vi "Shift GPS Output.vi"(1 "GPS Input":cluster{"X pos":i32, "Y pos":i32, "Heading":dbl}) -> (0 "GPS Output":cluster{"X pos":i32, "Y pos":i32, "Heading":dbl})   [LabVIEW 2014]
panel:
  out "Abs Angle":dbl
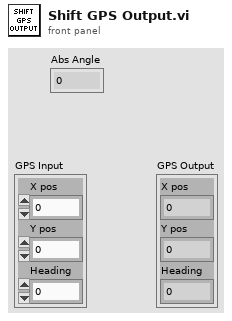
[diagram p1: front panel]
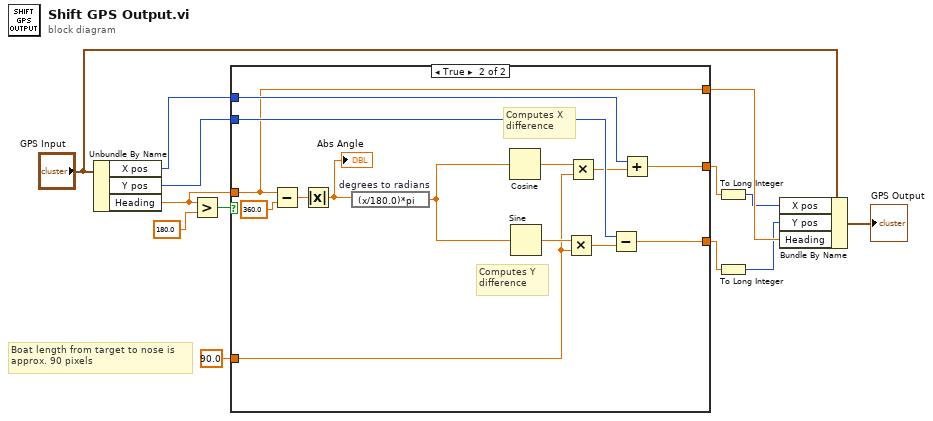
[diagram p0: block diagram]
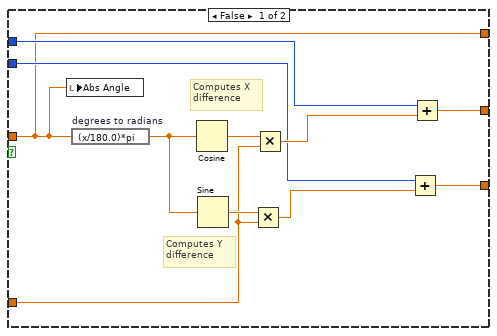
[diagram p2: hidden frame]
diagram:
  # "Boat length from target to nose is \napprox. 90 pixels"
  n1 = Unbundle By Name("GPS Input") -> ("X pos"=w11:i32, "Y pos"=w10:i32, "Heading"=w8:dbl)
  n2 = Greater?(x=w8, y=180.0) -> (0:w12:bool)
  n3 = case shown="True" w12 {
    tunnel: w11 -> [w20 w33]
    tunnel: w10 -> [w18 w32]
    tunnel: 90.0 -> [w22 w34]
    tunnel: w8 -> [w15 w29]
    tunnel: [w17 w31] -> w7
    tunnel: [w16 w30] -> w6
    tunnel: [w15 w29] -> w4
    frame False {
      # "Computes Y \ndifference"
      # "Computes X \ndifference"
      n4 = local write "Abs Angle"(w15) -> ()
      n5 = expression code="(x/180.0)*pi" "degrees to radians"(w15) -> (w14:dbl)
      n6 = Cosine(x=w14) -> (cos(x)=w24:dbl)
      n7 = Sine(x=w14) -> (sin(x)=w23:dbl)
      n8 = Multiply(x=w23, y=w22) -> (x*y=w19:dbl)
      n9 = Multiply(x=w24, y=w22) -> (x*y=w21:dbl)
      n10 = Add(x=w18, y=w19) -> (x+y=w16:dbl)
      n11 = Add(x=w20, y=w21) -> (x+y=w17:dbl)
    }
    frame True {
      # "Computes Y \ndifference"
      # "Computes X \ndifference"
      n12 = Subtract(x=w29, y=360.0) -> (x-y=w37:dbl)
      n13 = Absolute Value(x=w37) -> (abs(x)=w26:dbl)
      "Abs Angle" <- w26
      n14 = expression code="(x/180.0)*pi" "degrees to radians"(w26) -> (w25:dbl)
      n15 = Cosine(x=w25) -> (cos(x)=w36:dbl)
      n16 = Sine(x=w25) -> (sin(x)=w35:dbl)
      n17 = Multiply(x=w35, y=w34) -> (x*y=w27:dbl)
      n18 = Multiply(x=w36, y=w34) -> (x*y=w28:dbl)
      n19 = Subtract(x=w32, y=w27) -> (x-y=w30:dbl)
      n20 = Add(x=w33, y=w28) -> (x+y=w31:dbl)
    }
  }
  n21 = To Long Integer(number=w7) -> (32bit integer=w3:i32)
  n22 = To Long Integer(number=w6) -> (32bit integer=w2:i32)
  n23 = Bundle By Name(cluster="GPS Input", "X pos"=w3, "Y pos"=w2, "Heading"=w4) -> (→"GPS Output":cluster{"X pos":i32, "Y pos":i32, "Heading":dbl})
